vi "Autoscale Write.vi"(4 "error in (no error)":errorcluster, 5 "Value":u8, 6 "Container State":T2, 7 "Display State In":T1) -> (0 "error out":errorcluster, 3 "Display State Out":T1)   [LabVIEW 2013, in "Multivalue Buffer.xctl"]
uses:
  Multivalue Buffer.xctl
  <vilib>/_xctls/Container State.ctl
  MultiVal State.ctl
  <vilib>/_xctls/XControlSupport.lvlib
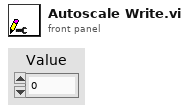
[diagram p1: front panel]
types:
  T1 = typedef "Multivalue Buffer.xctl/MultiVal State.ctl" = cluster{"History":i32, "Size":cluster{"Height":i32, "Width":i32}, "axis label":string, "Graph":refnum<vi>}
  T2 = typedef "XControlSupport.lvlib/Container State.ctl" = cluster{"Indicator?":bool, "Run Mode?":bool, " Refnum":refnum<vi>}
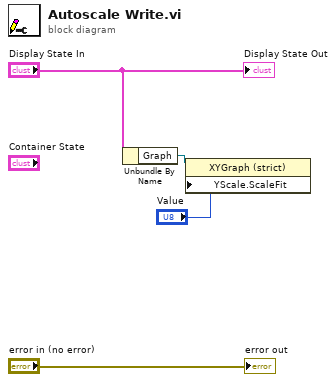
[diagram p0: block diagram]
diagram:
  n1 = Unbundle By Name("Display State In") -> ("Graph"=w2:refnum<vi>)
  n2 = property class="XYGraph (strict)"(reference=w2, "YScale.ScaleFit"="Value") -> ()  [unwired: 1 in, 2 out]
  "error out" <- "error in (no error)"
  "Display State Out" <- "Display State In"
